vi "Test Worker Process Job Broadcasts Status.vi"(8 "error in (no error)":errorcluster, 11 "Worker Test in":refnum<class "Worker Test.lvclass">) -> (0 "error out":errorcluster, 3 "Worker Test out":refnum<class "Worker Test.lvclass">)   [LabVIEW 2020, in "Worker Test.lvclass"]
uses:
  Worker Test.lvclass
  C:/Program Files (x86)/National Instruments/LabVIEW 2020/vi.lib/Asteme/LUnit/Test Case.lvclass
  Processes/People/Workers/Worker/Worker.lvclass
  C:/Program Files (x86)/National Instruments/LabVIEW 2020/vi.lib/Asteme/Triarc Framework/Process/Process.lvclass
  <vilib>/Asteme/Triarc Framework/Process/Process.lvclass/Process.ctl
  <vilib>/Asteme/LUnit/Test Case.lvclass/Test Case.ctl
  <vilib>/Asteme/LUnit/LUnit Assertion Result.lvclass/LUnit Assertion Result.ctl
  <vilib>/Asteme/Triarc Framework Test Suite/Support/Execution timer.vi
  <vilib>/Asteme/Triarc Framework/Process/Private/SubVIs/Wait for finish.vi
  <vilib>/Asteme/Triarc Framework/Process/Protected/Messaging/Enqueue Message.vi
  <vilib>/Asteme/Triarc Framework/Process/Private/SubVIs/Set Lifecycle State.vi
  <vilib>/Asteme/Triarc Framework/Process/Public/Lifecycle/Get Lifecycle State.vi
  <vilib>/Asteme/LUnit/Palette/Pass If.vi
  <vilib>/Asteme/LUnit/Set Assertion Type.vi
  <vilib>/Asteme/LUnit/Add test result.vi
  <vilib>/Asteme/LUnit/LUnit Get Test Case.vi
  <vilib>/Asteme/LUnit/Assertion Result/LUnit Get Test Name.vi
  <vilib>/Asteme/LUnit/LUnit Write Message.vi
  <vilib>/Asteme/LUnit/LUnit Write Description.vi
  <vilib>/Asteme/LUnit/LUnit Write Skipped.vi
  <vilib>/Utility/error.llb/Clear Errors.vi
  <vilib>/Asteme/LUnit/Palette/Fail.vi
  <vilib>/Asteme/LUnit/Palette/Pass.vi
  <vilib>/Asteme/LUnit/LUnit Write Assertion Type.vi
  <vilib>/Asteme/LUnit/Read Test Case Name.vi
  <vilib>/Asteme/LUnit/LUnit Write Passed.vi
  <vilib>/Asteme/Triarc Framework Test Suite/Support/Event Helpers/Dequeue Event Message.vi
  <vilib>/Utility/error.llb/Error Cluster From Error Code.vi
  <vilib>/Asteme/LUnit/LUnit Assertion Result.lvclass
  <vilib>/Asteme/Triarc Framework/Process/Process.lvclass
  <vilib>/Asteme/LUnit/Test Case.lvclass
  <vilib>/Asteme/Triarc Framework/Broadcast Event Helpers/Broadcast Event Helpers.lvlib
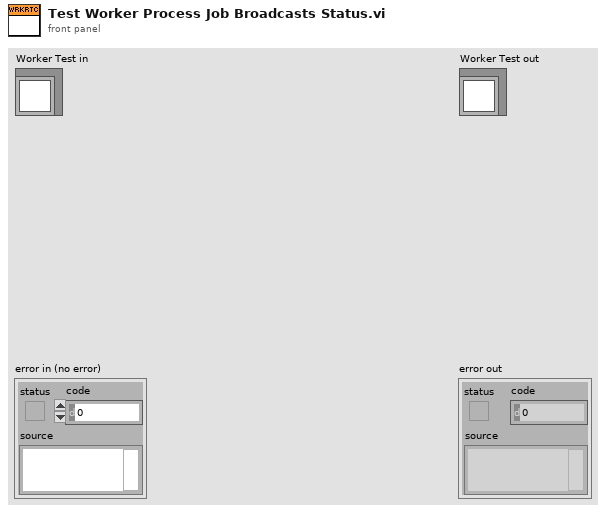
[diagram p1: front panel]
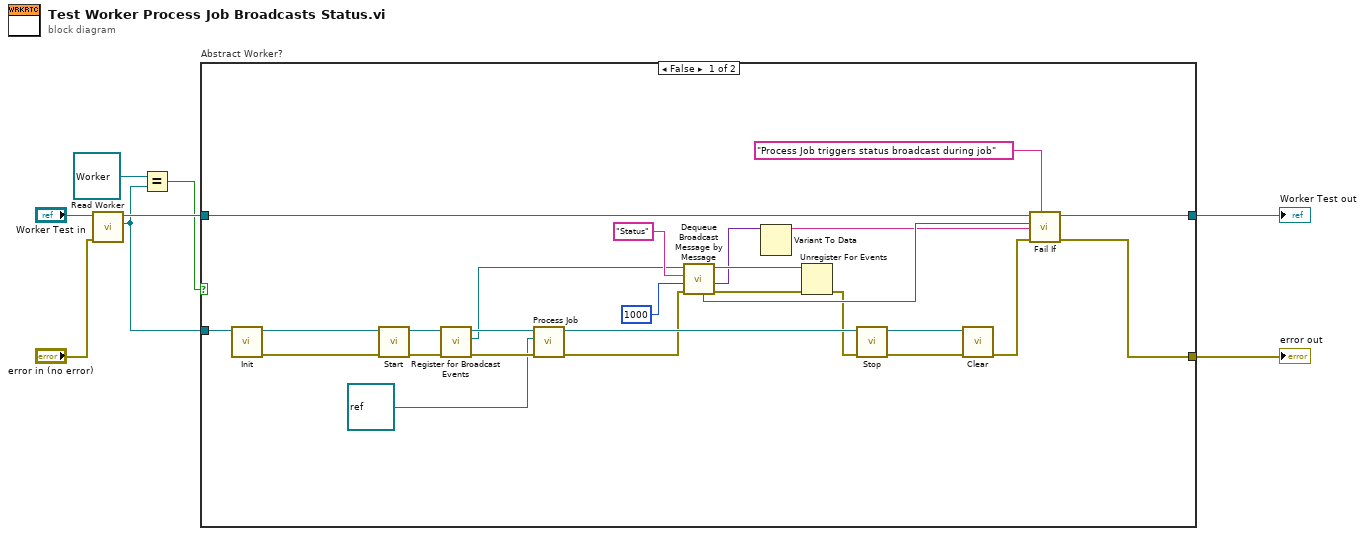
[diagram p0: block diagram]
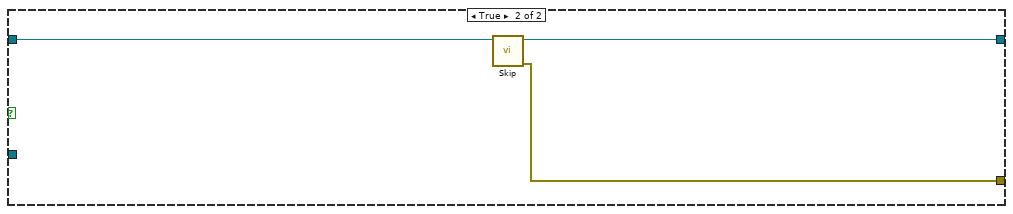
[diagram p2: hidden frame]
diagram:
  n1 = call "Read Worker.vi"("error in (no error)"="error in (no error)", "Worker Test in"="Worker Test in") -> ("Worker"=w2:refnum<class "Worker.lvclass">, "Worker Test out"=w5:refnum<class "Worker Test.lvclass">)  [unwired: 7 in, 1 out]
  n2 = Equal?(x=refnum<class "Worker.lvclass"> refnum ("Worker"), y=w2) -> (x = y?=w1:bool)
  n3 = case "Abstract Worker?" shown="False" w1 {
    tunnel: [w28 w35] -> w6
    tunnel: w5 -> [w27 w37]
    tunnel: [w17 w36] -> w4
    tunnel: w2 -> [w19 _]
    frame False {
      n4 = call-dynamic "Init.vi"("View In"=w19) -> ("error out"=w34:errorcluster, "View Out"=w31:refnum<class "Worker.lvclass">)  [unwired: 9 in]
      n5 = call <vilib>:"Start.vi"("error in (no error)"=w34, "Process In"=w31) -> ("error out"=w30:errorcluster, "Process Out"=w24:refnum<class "Worker.lvclass">)  [unwired: 8 in]
      n6 = call <vilib>:"Register for Broadcast Events.vi"("error in (no error)"=w30, "Process In"=w24) -> ("error out"=w25:errorcluster, "Event Registration Refnum Out"=w9:refnum<event-registration>, "Process Out"=w23:refnum<class "Worker.lvclass">)  [unwired: 7 in]
      n7 = call-dynamic "Process Job.vi"("error in (no error)"=w25, "Job"=refnum<class> refnum ("Task"), "Worker In"=w23) -> ("error out"=w21:errorcluster, "Worker Out"=w22:refnum<class "Worker.lvclass">)  [unwired: 7 in]
      n8 = call <vilib>:"Dequeue Broadcast Message by Message.vi"("error in (no error)"=w21, "Timeout (-1)"=1000, "Message"="Status", "Event Registration Refnum"=w9) -> ("error out"=w13:errorcluster, "Message Data"=w11:variant, "Event Registration Refnum Out"=w14:refnum<event-registration>, "Timed Out?"=w18:bool)  [unwired: 3 in, 1 out]
      n9 = Variant To Data(Variant=w11) -> (data=w10:string)  [unwired: 2 in, 1 out]
      n10 = Unregister For Events(event registration refnum=w14, error in=w13) -> (error out=w16:errorcluster)
      n11 = call <vilib>:"Stop.vi"("error in (no error)"=w16, "Process In"=w22) -> ("error out"=w32:errorcluster, "Process Out"=w33:refnum<class "Worker.lvclass">)  [unwired: 7 in, 1 out]
      n12 = call-dynamic "Clear.vi"("error in (no error)"=w32, "View In"=w33) -> ("error out"=w29:errorcluster)  [unwired: 9 in]
      n13 = call <vilib>:"Fail If.vi"("Description"="Process Job triggers status broadcast during job", "error in (no error)"=w29, "Message"=w10, "Fail?"=w18, "Test Case In"=w27) -> ("error out"=w28:errorcluster, "Test Case Out"=w17:refnum<class "Worker Test.lvclass">)  [unwired: 5 in]
    }
    frame True {
      n14 = call <vilib>:"Skip.vi"("Test Case In"=w37) -> ("error out"=w35:errorcluster, "Test Case Out"=w36:refnum<class "Worker Test.lvclass">)  [unwired: 9 in]
    }
  }
  "error out" <- w6
  "Worker Test out" <- w4
